vi "AR-Build-Axis-position-speed-graph.vi"(6 "Select":bool, 7 "Action":enum16{"Init", "WR", "RD"}(ring), 9 "error in (no error)":errorcluster, 10 "Loop time":u32, 11 "X Pos":dbl) -> (3 "Pos/Speed":cluster{u32[], dbl[]}(graph) caption="XY Graph - Light")   [LabVIEW 2021]
uses:
  <vilib>/Analysis/3filter.llb/Filter Passband Type.ctl
  <vilib>/Analysis/3filter.llb/Butterworth Filter (DBL).vi
  <vilib>/Analysis/NI_AALBase.lvlib
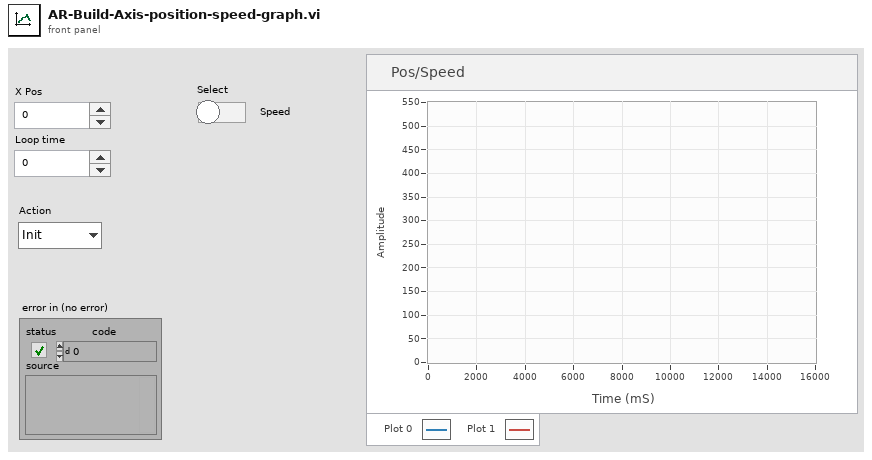
[diagram p1: front panel]
types:
  T1 = typedef "NI_AALBase.lvlib/Filter Passband Type.ctl" = enum32{"Lowpass", "Highpass", "Bandpass", "Bandstop"}
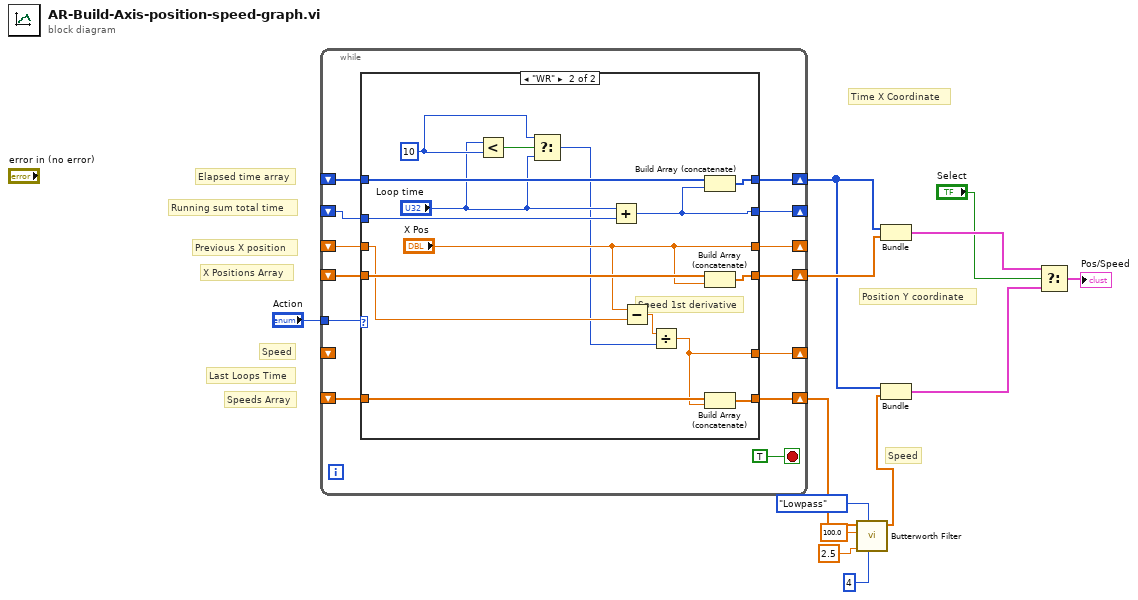
[diagram p0: block diagram]
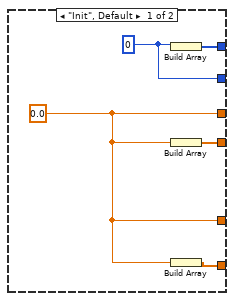
[diagram p2: hidden frame]
diagram:
  # "Speeds Array"
  # "Last Loops Time"
  # "Speed"
  # "X Positions Array"
  # "Previous X position"
  # "Running sum total time"
  # "Elapsed time array"
  # "Speed"
  # "Position Y coordinate"
  # "Time X Coordinate"
  n1 = while {
    tunnel: "Action" -> [w25]
    shift-right: [w23] -> _
    shift-left: _ -> [w22]
    shift-right: [w24] -> _
    shift-left: _ -> [w18]
    shift-right: [w21] -> w11
    shift-left: _ -> [w14]
    shift-right: [w20] -> w12
    shift-left: _ -> [w19]
    shift-right: [w17] -> _
    shift-left: _ -> [_]
    shift-right: [w16] -> w6
    shift-left: _ -> [w15]
    stop <- TRUE stop-if-true
    n2 = case shown="\"WR\"" w25 {
      tunnel: [w28 "X Pos"] -> w24
      tunnel: [w27 w45] -> w23
      tunnel: w22 -> [_ w36]
      tunnel: [w31 w46] -> w21
      tunnel: [w30 w44] -> w20
      tunnel: w14 -> [_ w47]
      tunnel: w19 -> [_ w43]
      tunnel: w18 -> [_ w41]
      tunnel: [w28 w37] -> w17
      tunnel: [w29 w39] -> w16
      tunnel: w15 -> [_ w38]
      frame "Init", Default {
        w27 = u32 0
        w28 = 0.0 ("X Pos")
        n3 = Build Array(w27) -> (w31:u32[])
        n4 = Build Array(w28) -> (w30:dbl[])
        n5 = Build Array(w28) -> (w29:dbl[])
      }
      frame "WR" {
        w34 = u32 10 ("y")
        # "Speed 1st derivative"
        n6 = Less?(x="Loop time", y=w34) -> (x < y?=w35:bool)
        n7 = Select(t=w34, s=w35, f="Loop time") -> (s? t:f=w32:u32)
        n8 = Add(x="Loop time", y=w36) -> (x+y=w45:u32)
        n9 = Subtract(x="X Pos", y=w41) -> (x-y=w40:dbl)
        n10 = Divide(x=w40, y=w32) -> (x/y=w37:dbl)
        n11 = Build Array (concatenate)(w47, w45) -> (w46:u32[])
        n12 = Build Array (concatenate)(w43, "X Pos") -> (w44:dbl[])
        n13 = Build Array (concatenate)(w38, w37) -> (w39:dbl[])
      }
    }
  }
  n14 = call-poly <vilib>:"Butterworth Filter.vi"("order"=4, "filter type"=Filter_Passband_Type."Lowpass", "low cutoff freq: fl"=2.5 ("high cutoff freq: fh"), "sampling freq: fs"=100.0, "X"=w6) -> ("Filtered X"=w3:dbl[])  [unwired: 3 in, 1 out]
  n15 = Bundle(w11, w12) -> (w10:cluster{u32[], dbl[]})  [unwired: 1 in]
  n16 = Bundle(w11, "Filtered X"=w3) -> (w9:cluster{u32[], "Filtered X":dbl[]})  [unwired: 1 in]
  n17 = Select(t=w10, s="Select", f=w9) -> (s? t:f=→"Pos/Speed":cluster{u32[], "Filtered X":dbl[]})
